vi "Build.vi"(8 "error in (no error)":errorcluster, 10 "Concrete Send Builder in":refnum<class "Concrete Send Builder.lvclass">, 11 "Scripter in":refnum<class "Message Scripter.lvclass">) -> (0 "error out":errorcluster, 2 "Concrete Send Builder out":refnum<class "Concrete Send Builder.lvclass">, 3 "Scripter out":refnum<class "Message Scripter.lvclass">)   [LabVIEW 2020, in "Message Maker.lvlib" / "Concrete Send Builder.lvclass"]
uses:
  Concrete Send Builder.lvclass
  Message Maker.lvlib
  Message Scripter/Message Scripter.lvclass
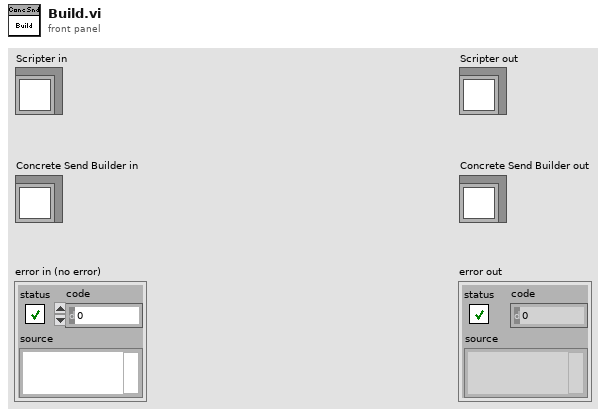
[diagram p1: front panel]
types:
  T1 = enum16{"Invalid Wire Rule", "Required", "Recommended", "Optional", "Dynamic Dispatch"}[]
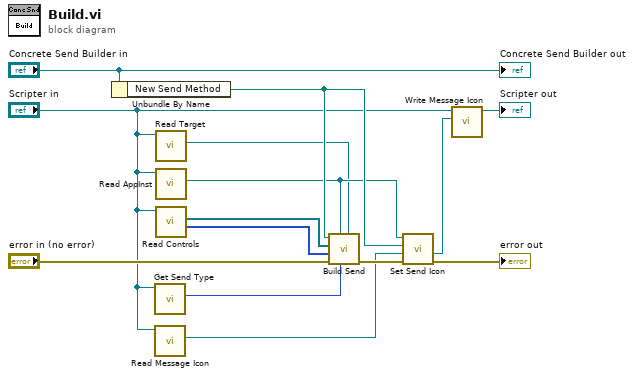
[diagram p0: block diagram]
diagram:
  n1 = Unbundle By Name("Concrete Send Builder in") -> ("New Send Method"=w14:path)
  n2 = call-dynamic "Get Send Type.vi"("Message Scripter in"="Scripter in") -> ("Send Type"=w12:enum16{"Concrete", "Abstract"})  [unwired: 10 in]
  n3 = call-dynamic "Read Message Icon.vi"("Message Scripter in"="Scripter in") -> ("Message Icon"=w7:refnum<class "Icon.lvclass">)  [unwired: 10 in]
  n4 = call "Read Target.vi"("Message Scripter in"="Scripter in") -> ("Target"=w1:refnum<vi>)  [unwired: 10 in]
  n5 = call "Read AppInst.vi"("Message Maker in"="Scripter in") -> ("AppInst"=w4:refnum<vi>)  [unwired: 10 in]
  n6 = call "Read Controls.vi"("Message Scripter in"="Scripter in") -> ("Wiring Rules"=w11:T1, "Controls[]"=w10:refnum<vi>[])  [unwired: 9 in]
  n7 = call "Build Send.vi"("Target"=w1, "Class Type"=w12, "AppInst"=w4, "error in (no error)"="error in (no error)", "Wiring Rules"=w11, "Controls"=w10, "Send Method path"=w14) -> ("error out"=w9:errorcluster)  [unwired: 4 in]
  n8 = call "Set Send Icon.vi"("error in (no error)"=w9, "Icon in"=w7, "Send Method path"=w14, "AppInst"=w4) -> ("error out"=→"error out":errorcluster, "Icon out"=w5:refnum<class "Icon.lvclass">)  [unwired: 6 in]
  n9 = call-dynamic "Write Message Icon.vi"("Message Icon"=w5, "Message Scripter in"="Scripter in") -> ("Message Scripter out"=→"Scripter out":refnum<class "Message Scripter.lvclass">)  [unwired: 9 in]
  "Concrete Send Builder out" <- "Concrete Send Builder in"
